vi "8ch_SigProcessing(SubVI).vi"(1 "Coefficient":dbl[](array[numeric]), 2 "decimating factor":i32=1 caption="부분제거 전환율", 3 "Carrier":dbl[](array[numeric]), 4 "8ch_INPUT":waveform(dbl)[](array[waveform])) -> (0 "8ch_OUTPUT":dbl[][](array[numeric]))   [LabVIEW 2017]
uses:
  <vilib>/Analysis/2dsp.llb/Decimate (single shot, DBL).vi
  <vilib>/Analysis/3filter.llb/FIR Filter (DBL).vi
  <vilib>/Analysis/NI_AALBase.lvlib
  <vilib>/Analysis/NI_AALPro.lvlib
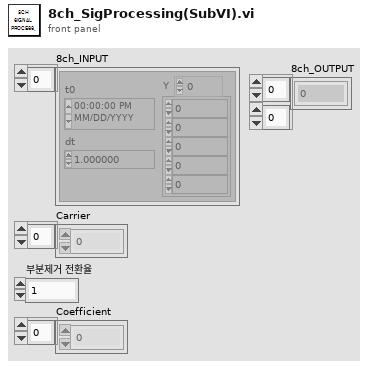
[diagram p1: front panel]
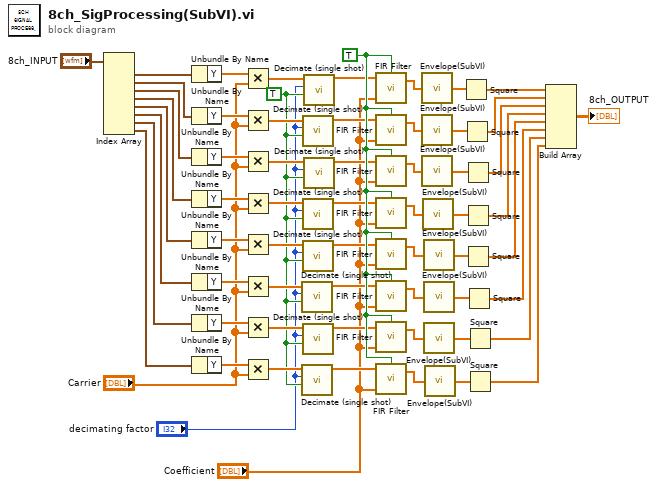
[diagram p0: block diagram]
diagram:
  w14 = TRUE ("averaging")
  w63 = TRUE ("init/cont (init:F)")
  n1 = Index Array(array="8ch_INPUT") -> (element #1=w62:waveform(dbl), element #2=w61:waveform(dbl), element #3=w60:waveform(dbl), element #4=w59:waveform(dbl), element #5=w58:waveform(dbl), element #6=w57:waveform(dbl), element #7=w56:waveform(dbl), element #8=w55:waveform(dbl))  [unwired: 8 in]
  n2 = Unbundle By Name(w62) -> ("Y"=w54:dbl[])
  n3 = Unbundle By Name(w61) -> ("Y"=w53:dbl[])
  n4 = Unbundle By Name(w60) -> ("Y"=w52:dbl[])
  n5 = Unbundle By Name(w59) -> ("Y"=w51:dbl[])
  n6 = Unbundle By Name(w58) -> ("Y"=w50:dbl[])
  n7 = Unbundle By Name(w57) -> ("Y"=w49:dbl[])
  n8 = Unbundle By Name(w56) -> ("Y"=w48:dbl[])
  n9 = Unbundle By Name(w55) -> ("Y"=w47:dbl[])
  n10 = Multiply(x=w54, y="Carrier") -> (x*y=w29:dbl[])
  n11 = Multiply(x=w53, y="Carrier") -> (x*y=w28:dbl[])
  n12 = Multiply(x=w52, y="Carrier") -> (x*y=w27:dbl[])
  n13 = Multiply(x=w51, y="Carrier") -> (x*y=w26:dbl[])
  n14 = Multiply(x=w50, y="Carrier") -> (x*y=w25:dbl[])
  n15 = Multiply(x=w49, y="Carrier") -> (x*y=w24:dbl[])
  n16 = Multiply(x=w48, y="Carrier") -> (x*y=w23:dbl[])
  n17 = Multiply(x=w47, y="Carrier") -> (x*y=w22:dbl[])
  n18 = call-poly <vilib>:"Decimate (single shot).vi"("averaging"=w14, "decimating factor"="decimating factor", "X"=w24) -> ("Decimated Array"=w17:dbl[])  [unwired: 7 in, 1 out]
  n19 = call-poly <vilib>:"Decimate (single shot).vi"("averaging"=w14, "decimating factor"="decimating factor", "X"=w22) -> ("Decimated Array"=w15:dbl[])  [unwired: 7 in, 1 out]
  n20 = call-poly <vilib>:"Decimate (single shot).vi"("averaging"=w14, "decimating factor"="decimating factor", "X"=w28) -> ("Decimated Array"=w21:dbl[])  [unwired: 7 in, 1 out]
  n21 = call-poly <vilib>:"Decimate (single shot).vi"("averaging"=w14, "decimating factor"="decimating factor", "X"=w26) -> ("Decimated Array"=w19:dbl[])  [unwired: 7 in, 1 out]
  n22 = call-poly <vilib>:"Decimate (single shot).vi"("averaging"=w14, "decimating factor"="decimating factor", "X"=w25) -> ("Decimated Array"=w18:dbl[])  [unwired: 7 in, 1 out]
  n23 = call-poly <vilib>:"Decimate (single shot).vi"("averaging"=w14, "decimating factor"="decimating factor", "X"=w23) -> ("Decimated Array"=w16:dbl[])  [unwired: 7 in, 1 out]
  n24 = call-poly <vilib>:"Decimate (single shot).vi"("averaging"=w14, "decimating factor"="decimating factor", "X"=w29) -> ("Decimated Array"=w30:dbl[])  [unwired: 7 in, 1 out]
  n25 = call-poly <vilib>:"Decimate (single shot).vi"("averaging"=w14, "decimating factor"="decimating factor", "X"=w27) -> ("Decimated Array"=w20:dbl[])  [unwired: 7 in, 1 out]
  n26 = call-poly <vilib>:"FIR Filter.vi"("init/cont (init:F)"=w63, "FIR Coefficients"="Coefficient", "X"=w30) -> ("Filtered X"=w46:dbl[])  [unwired: 1 in, 1 out]
  n27 = call-poly <vilib>:"FIR Filter.vi"("init/cont (init:F)"=w63, "FIR Coefficients"="Coefficient", "X"=w21) -> ("Filtered X"=w45:dbl[])  [unwired: 1 in, 1 out]
  n28 = call-poly <vilib>:"FIR Filter.vi"("init/cont (init:F)"=w63, "FIR Coefficients"="Coefficient", "X"=w20) -> ("Filtered X"=w44:dbl[])  [unwired: 1 in, 1 out]
  n29 = call-poly <vilib>:"FIR Filter.vi"("init/cont (init:F)"=w63, "FIR Coefficients"="Coefficient", "X"=w19) -> ("Filtered X"=w43:dbl[])  [unwired: 1 in, 1 out]
  n30 = call-poly <vilib>:"FIR Filter.vi"("init/cont (init:F)"=w63, "FIR Coefficients"="Coefficient", "X"=w18) -> ("Filtered X"=w42:dbl[])  [unwired: 1 in, 1 out]
  n31 = call-poly <vilib>:"FIR Filter.vi"("init/cont (init:F)"=w63, "FIR Coefficients"="Coefficient", "X"=w17) -> ("Filtered X"=w41:dbl[])  [unwired: 1 in, 1 out]
  n32 = call-poly <vilib>:"FIR Filter.vi"("init/cont (init:F)"=w63, "FIR Coefficients"="Coefficient", "X"=w16) -> ("Filtered X"=w40:dbl[])  [unwired: 1 in, 1 out]
  n33 = call-poly <vilib>:"FIR Filter.vi"("init/cont (init:F)"=w63, "FIR Coefficients"="Coefficient", "X"=w15) -> ("Filtered X"=w39:dbl[])  [unwired: 1 in, 1 out]
  n34 = call "Envelope(SubVI).vi"("x"=w46) -> ("Y"=w38:dbl[])
  n35 = call "Envelope(SubVI).vi"("x"=w45) -> ("Y"=w37:dbl[])
  n36 = call "Envelope(SubVI).vi"("x"=w44) -> ("Y"=w36:dbl[])
  n37 = call "Envelope(SubVI).vi"("x"=w43) -> ("Y"=w35:dbl[])
  n38 = call "Envelope(SubVI).vi"("x"=w42) -> ("Y"=w34:dbl[])
  n39 = call "Envelope(SubVI).vi"("x"=w41) -> ("Y"=w33:dbl[])
  n40 = call "Envelope(SubVI).vi"("x"=w40) -> ("Y"=w32:dbl[])
  n41 = call "Envelope(SubVI).vi"("x"=w39) -> ("Y"=w31:dbl[])
  n42 = Square(x=w38) -> (x^2=w13:dbl[])
  n43 = Square(x=w37) -> (x^2=w12:dbl[])
  n44 = Square(x=w36) -> (x^2=w11:dbl[])
  n45 = Square(x=w35) -> (x^2=w10:dbl[])
  n46 = Square(x=w34) -> (x^2=w9:dbl[])
  n47 = Square(x=w33) -> (x^2=w8:dbl[])
  n48 = Square(x=w32) -> (x^2=w7:dbl[])
  n49 = Square(x=w31) -> (x^2=w6:dbl[])
  n50 = Build Array(w13, w12, w11, w10, w9, w8, w7, w6) -> (→"8ch_OUTPUT":dbl[][])
